vi "5302GPIBCommCut.vi"(8 "error in (no error)":errorcluster, 9 "data string in":string, 11 "VISA Resource Name":refnum<visa-resource-name>) -> (0 "error out":errorcluster, 1 "data string out":string, 3 "VISA Resource Name Out":refnum<visa-resource-name>)   [LabVIEW 2015]
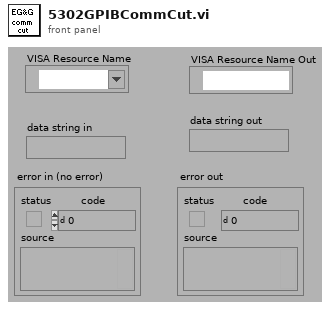
[diagram p1: front panel]
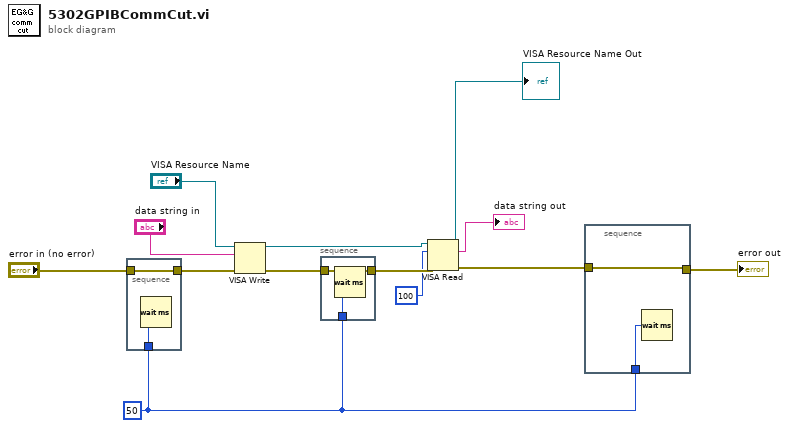
[diagram p0: block diagram]
diagram:
  w11 = 50
  n1 = stacked-sequence {
    tunnel: "error in (no error)" -> [w15]
    tunnel: [w15] -> w7
    tunnel: w11 -> [w14]
    frame #0 {
      n2 = Wait (ms)(milliseconds to wait=w14) -> ()  [unwired: 1 out]
    }
  }
  n3 = VISA Write(VISA resource name="VISA Resource Name", write buffer="data string in", error in (no error)=w7) -> (VISA resource name out=w3:refnum<visa-resource-name>, error out=w8:errorcluster)  [unwired: 1 out]
  n4 = stacked-sequence {
    tunnel: w8 -> [w17]
    tunnel: [w17] -> w9
    tunnel: w11 -> [w16]
    frame #0 {
      n5 = Wait (ms)(milliseconds to wait=w16) -> ()  [unwired: 1 out]
    }
  }
  n6 = VISA Read(VISA resource name=w3, byte count=u32 100 ("count"), error in (no error)=w9) -> (VISA resource name out=→"VISA Resource Name Out":refnum<visa-resource-name>, read buffer=→"data string out":string, error out=w10:errorcluster)  [unwired: 1 out]
  n7 = stacked-sequence {
    tunnel: [w19] -> w13
    tunnel: w10 -> [w19]
    tunnel: w11 -> [w18]
    frame #0 {
      n8 = Wait (ms)(milliseconds to wait=w18) -> ()  [unwired: 1 out]
    }
  }
  "error out" <- w13
